vi "Read Parent Stop Notifier.vi"(8 "error in (no error)":errorcluster, 11 "Node Actor in":refnum<class "Node Actor.lvclass">) -> (0 "error out":errorcluster, 1 "Stop":bool, 3 "Node Actor out":refnum<class "Node Actor.lvclass">)   [LabVIEW 2024, in "Node Actor.lvclass"]
uses:
  Node Actor.lvclass
  Node Actor.lvclass/Node Actor.ctl
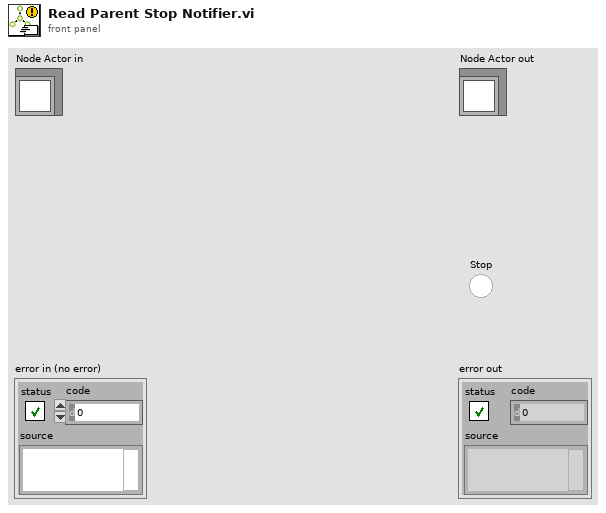
[diagram p1: front panel]
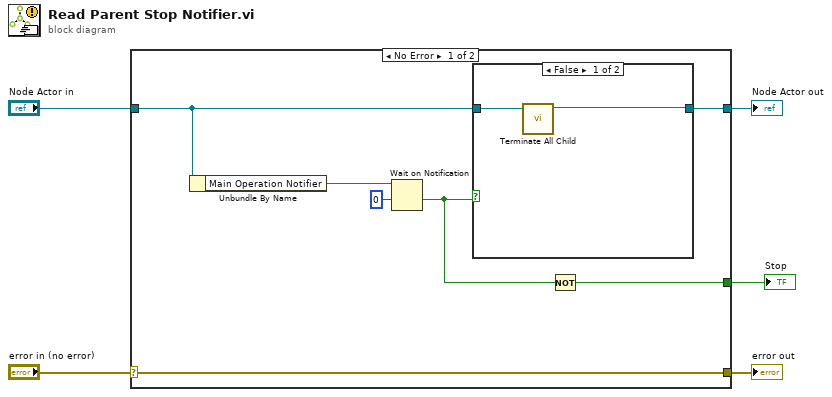
[diagram p0: block diagram]
diagram:
  n1 = case shown="No Error" "error in (no error)" {
    selector: "error in (no error)" -> [w12 w17]
    tunnel: [w12 w17] -> w4
    tunnel: [w8 w16] -> w2
    tunnel: "Node Actor in" -> [w9 w16]
    tunnel: [w6 _] -> w1
    frame No Error {
      n2 = Unbundle By Name(w9) -> ("Main Operation Notifier"=w11:refnum<notifier>)
      n3 = Wait on Notification(notifier=w11, timeout in ms (-1)=0) -> (timed out?=w7:bool)  [unwired: 2 in, 3 out]
      n4 = case shown="False" w7 {
        tunnel: w9 -> [w14 w15]
        tunnel: [w13 w15] -> w8
        frame False {
          n5 = call "Terminate All Child.vi"("Node Actor in"=w14) -> ("Node Actor out"=w13:refnum<class "Node Actor.lvclass">)  [unwired: 9 in, 1 out]
        }
        frame True {
        }
      }
      n6 = Not(x=w7) -> (.not. x?=w6:bool)
    }
    frame Error {
    }
  }
  "error out" <- w4
  "Node Actor out" <- w2
  "Stop" <- w1
